vi "function1.vi"(1 "y":dbl) -> (0 "x+y":dbl)   [LabVIEW 2012]
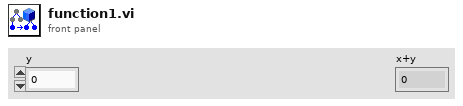
[diagram p1: front panel]
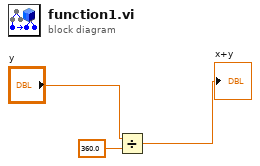
[diagram p0: block diagram]
diagram:
  n1 = Divide(x="y", y=360.0) -> (x/y=→"x+y":dbl)
